vi "AddLeft(SubVI).vi"(11 "Array in":i32[](array[numeric])) -> (1 "Score":i32, 2 "Array out":i32[](array[numeric]), 3 "tiles moved?":bool)   [LabVIEW 2020]
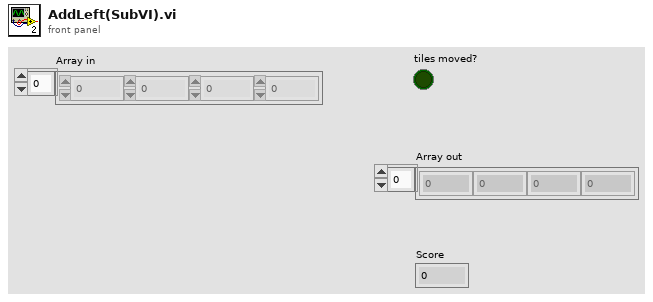
[diagram p1: front panel]
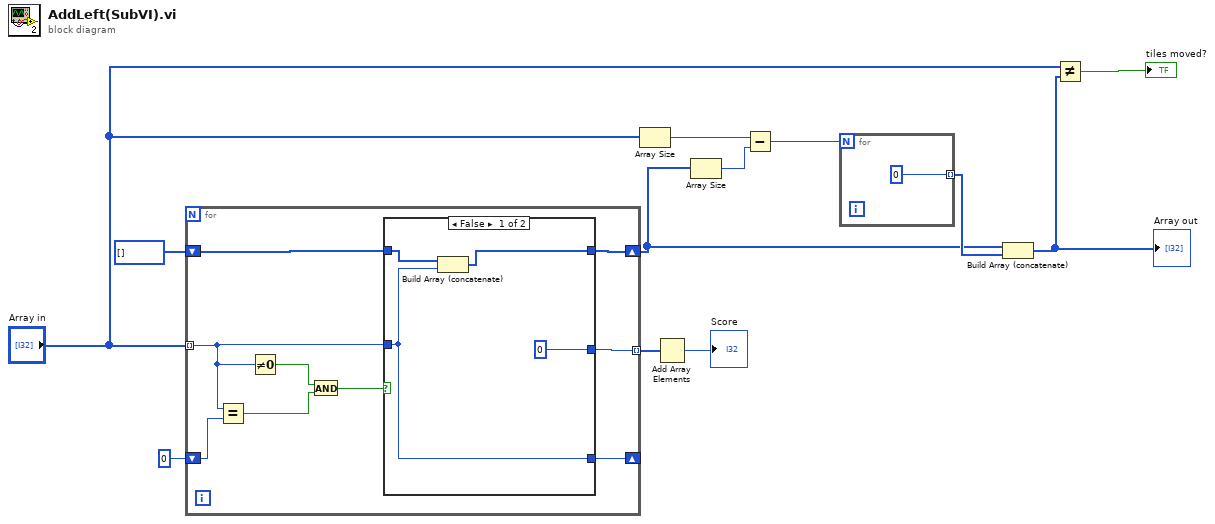
[diagram p0: block diagram]
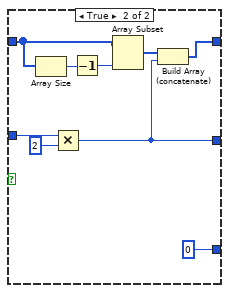
[diagram p2: hidden frame]
diagram:
  n1 = for {
    shift-right: [w14] -> w9
    shift-left: i32[] [] ("Array 3") -> [w21]
    tunnel: "Array in" -> [w16] mode=indexing
    shift-right: [w13] -> _
    shift-left: 0 -> [w17]
    tunnel: [w15] -> w3 mode=indexing
    n2 = Equal?(x=w16, y=w17) -> (x = y?=w19:bool)
    n3 = Not Equal To 0?(x=w16) -> (x != 0?=w20:bool)
    n4 = And(x=w20, y=w19) -> (x .and. y?=w18:bool)
    n5 = case shown="False" w18 {
      tunnel: w21 -> [w24 w30]
      tunnel: w16 -> [w23 w34]
      tunnel: [0 w28] -> w15
      tunnel: [w25 w27] -> w14
      tunnel: [w23 0] -> w13
      frame False {
        n6 = Build Array (concatenate)(w24, w23) -> (w25:i32[])
      }
      frame True {
        n7 = Array Size(array=w30) -> (size(s)=w32:i32)
        n8 = Multiply(x=w34, y=2) -> (x*y=w28:i32)
        n9 = Decrement(x=w32) -> (x-1=w31:i32)
        n10 = Array Subset(array=w30, length=w31) -> (w29:i32[])  [unwired: 1 in]
        n11 = Build Array (concatenate)(w29, w28) -> (w27:i32[])
      }
    }
  }
  n12 = Array Size(array="Array in") -> (size(s)=w6:i32)
  n13 = Add Array Elements(numeric array=w3) -> (sum=→"Score":i32)
  n14 = Array Size(array=w9) -> (size(s)=w5:i32)
  n15 = Subtract(x=w6, y=w5) -> (x-y=w7:i32)
  n16 = for {
    N: w7 -> [_]
    tunnel: [0] -> w10 mode=indexing
  }
  n17 = Build Array (concatenate)(w9, w10) -> (w11:i32[])
  "Array out" <- w11
  n18 = Not Equal?(x="Array in", y=w11) -> (x != y?=→"tiles moved?":bool)
